vi "monitoring_sys_final.vi"() -> ()   [LabVIEW 2023]
panel:
  in  "?":T1(tab)
  in  "?":bool
  out "Humidity [%]":dbl
  out "Temperture [C] 2":dbl
  out "Oxygen Level [%]":dbl
  out "?":bool
  out "Door's status 2":bool
  out "?":string
  out "string array 2":string[](array[string]) caption="Entry and Exit Data"
  out "Waiting for Message 2":bool
  in  "?":T2(tab)
  out "Pressure Gauge 130B":picture
  out "Glove Box Panel_001 130B":picture
  out "Glove Box Panel_011 130B":picture
  out "Glove Box Panel_002 130B":picture
  out "Glove Box Panel_022 130B":picture
  out "?":bool
  out "Door's status":bool
  out "Oxygen Level [%]":dbl
  out "Temperture [C]":dbl
  out "Humidity [%]":dbl
  out "Waiting for Message":bool
  out "?":string
  in  "?":bool
  out "string array":string[](array[string]) caption="Entry and Exit Data"
  in  "?":bool
  out "Humidity [%]  2":dbl
  out "Temperture [C] 3":dbl
  out "Oxygen Level [%]  2":dbl
  out "?":bool
  out "Waiting for Message 3":bool
  out "Message from Server":string
  out "Error Out":errorcluster caption="Error"
  out "Data from ESP32":dbl[](array[numeric])
  out "Error Out 2":errorcluster caption="Error 2"
  out "Error Out 3":errorcluster caption="Error"
  out "Data from ESP32 2":dbl[](array[numeric])
  out "Data from ESP32 3":dbl[](array[numeric])
  out "Message from Server 2":string
  out "Message from Server 3":string
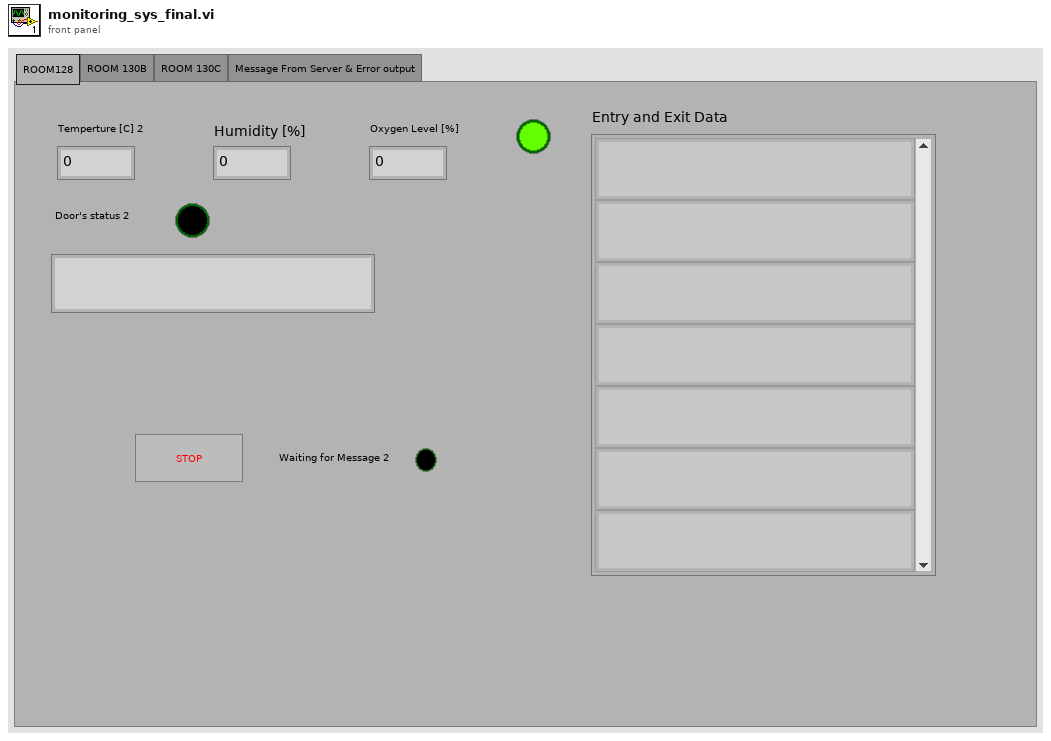
[diagram p1: front panel]
types:
  T1 = enum32{"ROOM128", "ROOM 130B", "ROOM 130C", "Message From Server & Error output"}
  T2 = enum32{"Liquid Nitrogen Tank gauge", "Glove Box 01 Control Panel", "Glove Box 01 Matchine Oil Level", "Glove Box 02 Control Panel", "Glove Box 02 Matchine Oil Level"}
  T3 = enum16{"Standard", "Buffered", "CRLF", "Immediate"}
  T4 = typedef "imagedata.ctl" = cluster{"image type":i32, "image depth":i32, "image":u8[], "mask":u8[], "colors":u32[], "Rectangle":cluster{"left":i16, "top":i16, "right":i16, "bottom":i16}}
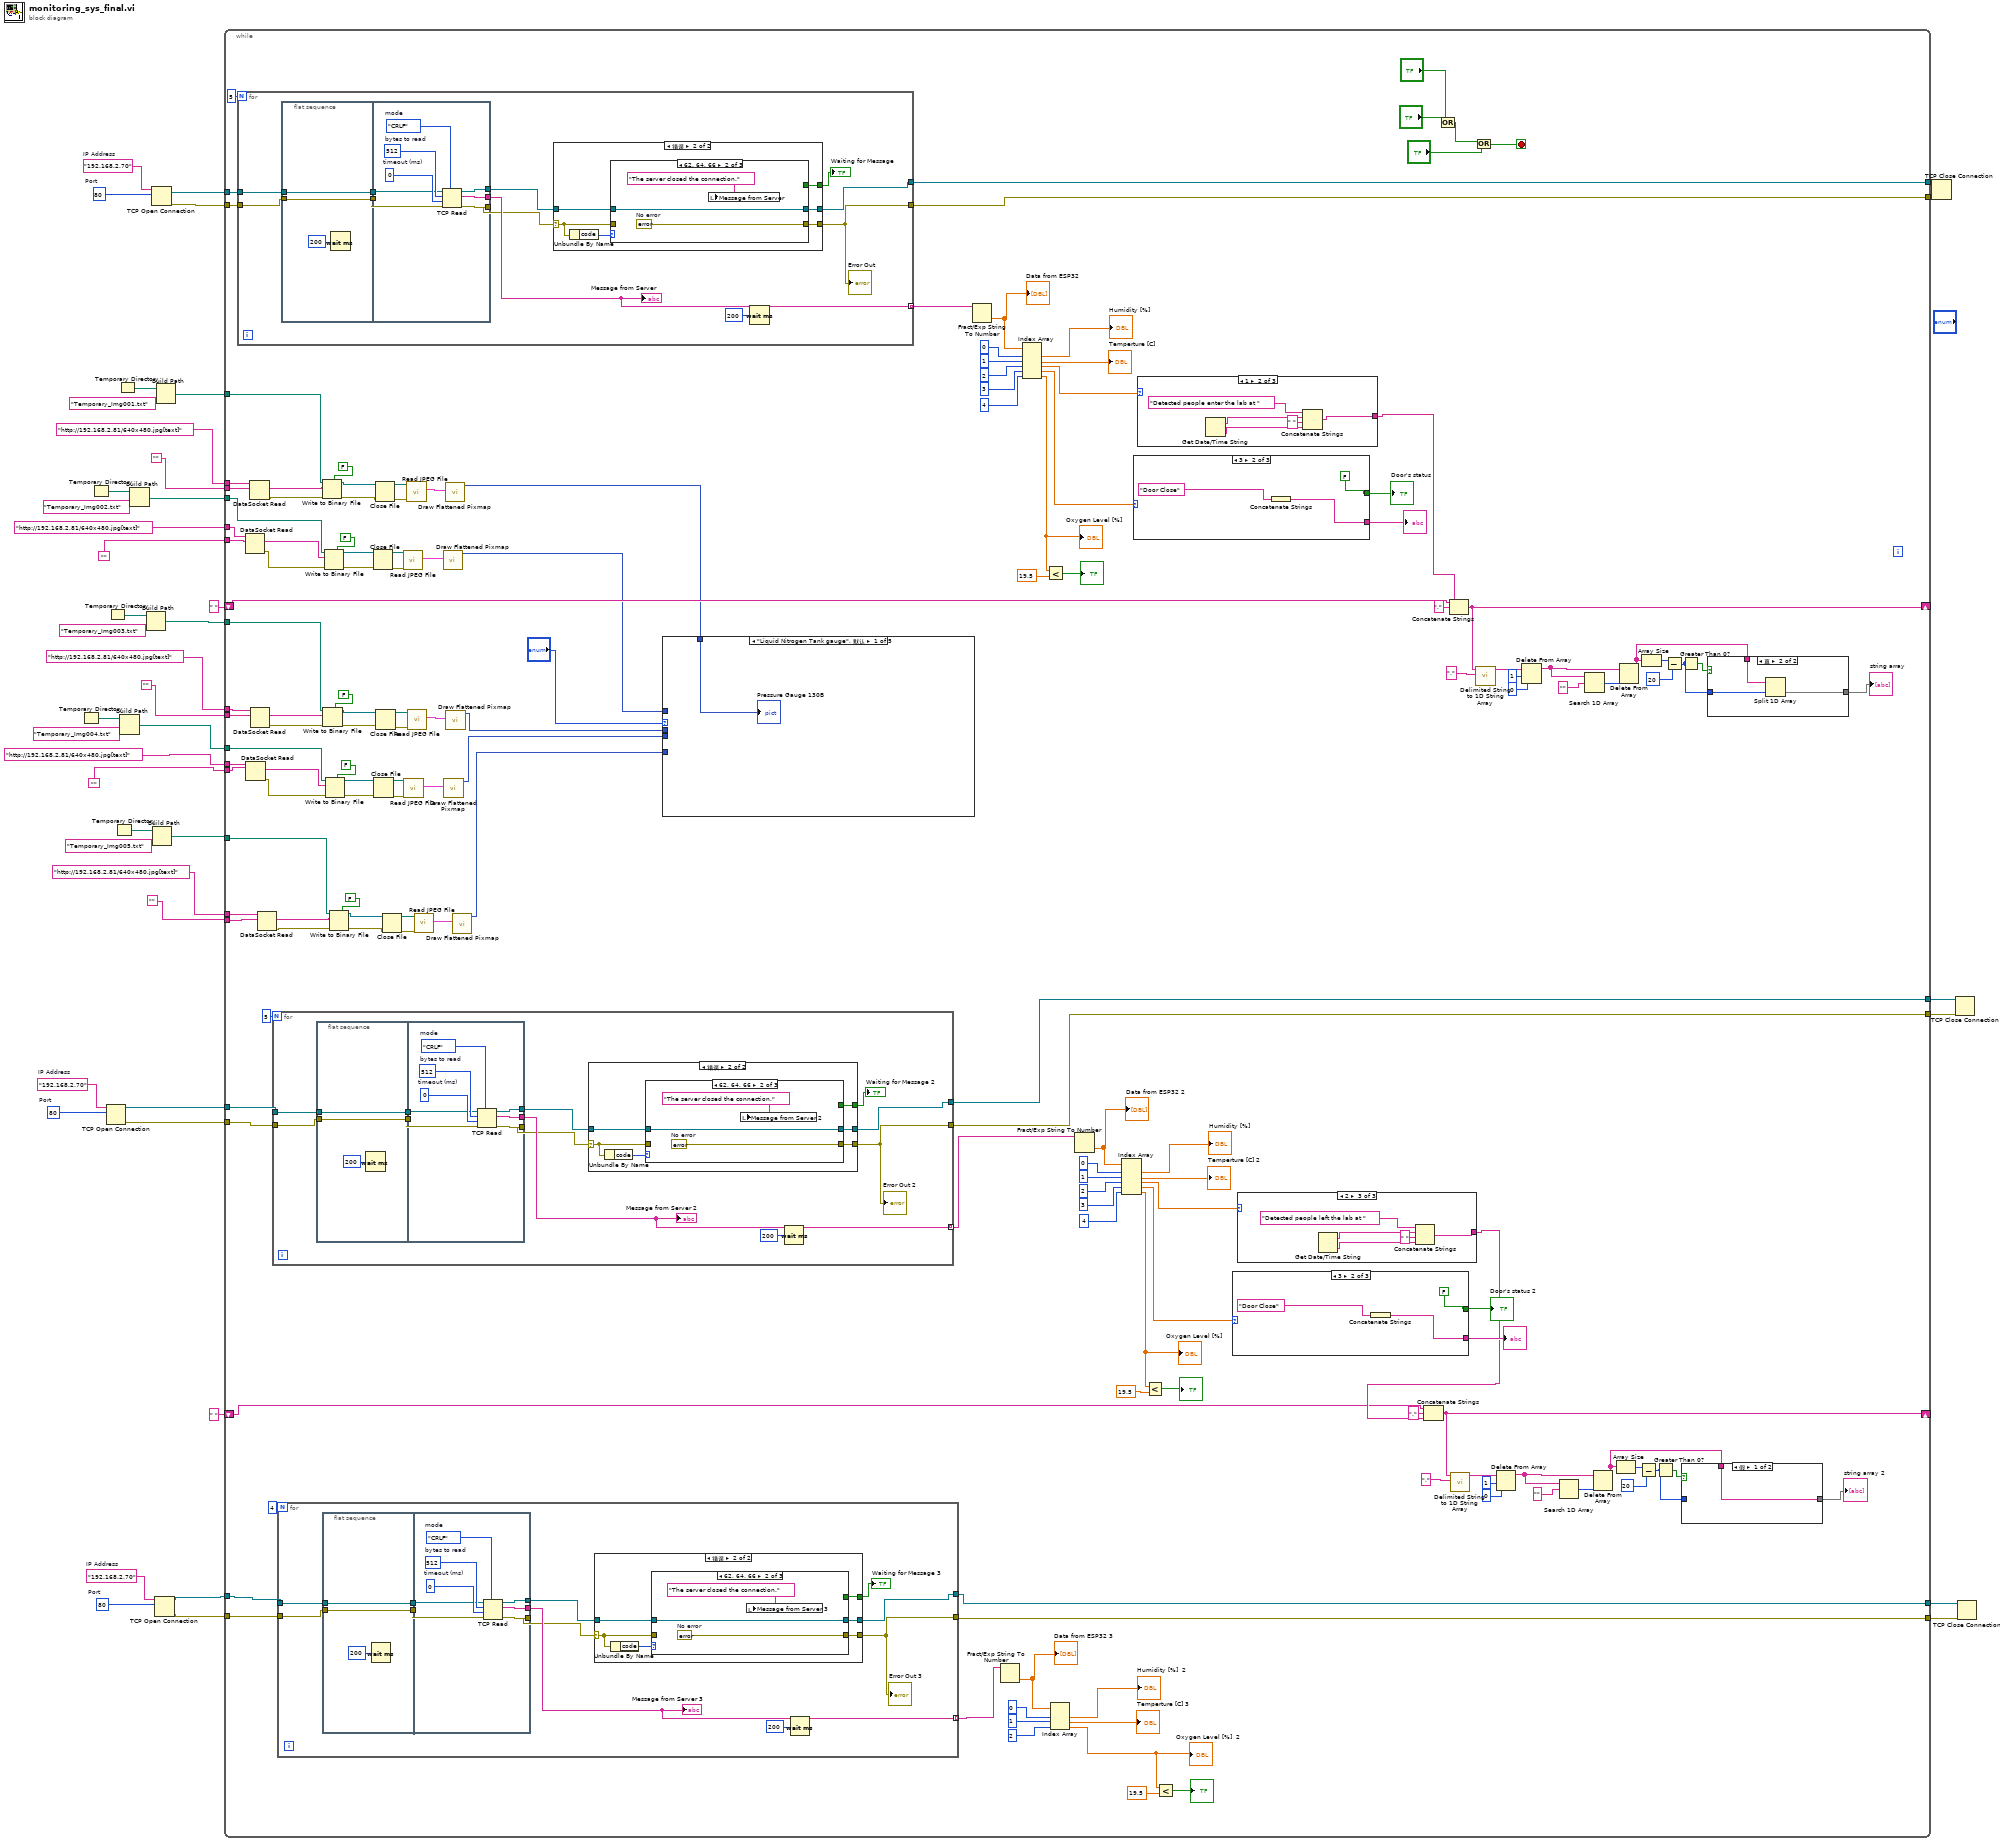
[diagram p0: block diagram]
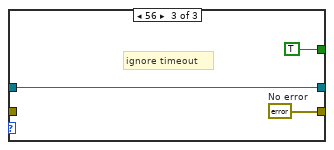
[diagram p4: hidden frame]
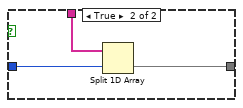
[diagram p5: hidden frame]
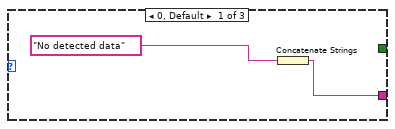
[diagram p6: hidden frame]
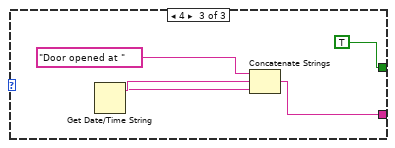
[diagram p7: hidden frame]
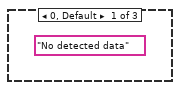
[diagram p8: hidden frame]
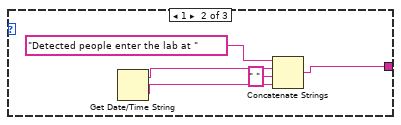
[diagram p9: hidden frame]
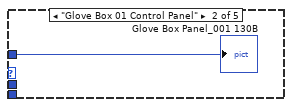
[diagram p10: hidden frame]
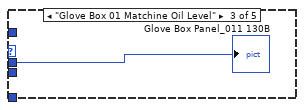
[diagram p11: hidden frame]
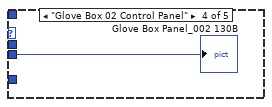
[diagram p12: hidden frame]
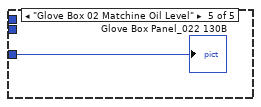
[diagram p13: hidden frame]
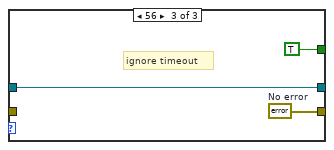
[diagram p16: hidden frame]
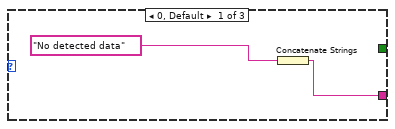
[diagram p18: hidden frame]
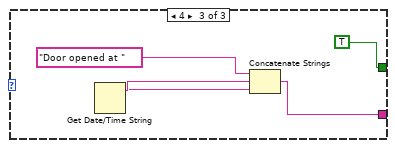
[diagram p19: hidden frame]
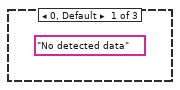
[diagram p20: hidden frame]
diagram:
  w7 = u16 80  # Port
  w8 = "192.168.2.70"  # IP Address
  w28 = u16 80  # Port
  w29 = "192.168.2.70"  # IP Address
  w44 = u16 80  # Port
  w45 = "192.168.2.70"  # IP Address
  n1 = Temporary Directory() -> (w23:path)
  n2 = Temporary Directory() -> (w32:path)
  n3 = TCP Open Connection(address=w29, remote port or service name=w28) -> (connection ID=w27:refnum<k5>, error out=w26:errorcluster)  [unwired: 3 in]
  n4 = Temporary Directory() -> (w25:path)
  n5 = Temporary Directory() -> (w15:path)
  n6 = Temporary Directory() -> (w35:path)
  n7 = Build Path(base path=w23, name or relative path="Temporary_Img004.txt") -> (appended path=w18:path)
  n8 = Build Path(base path=w32, name or relative path="Temporary_Img002.txt") -> (appended path=w30:path)
  n9 = Build Path(base path=w25, name or relative path="Temporary_Img003.txt") -> (appended path=w21:path)
  n10 = TCP Open Connection(address=w45, remote port or service name=w44) -> (connection ID=w43:refnum<k5>, error out=w42:errorcluster)  [unwired: 3 in]
  n11 = Build Path(base path=w15, name or relative path="Temporary_Img005.txt") -> (appended path=w13:path)
  n12 = TCP Open Connection(address=w8, remote port or service name=w7) -> (connection ID=w6:refnum<k5>, error out=w5:errorcluster)  [unwired: 3 in]
  n13 = Build Path(base path=w35, name or relative path="Temporary_Img001.txt") -> (appended path=w33:path)
  n14 = while {
    tunnel: w43 -> [w201]
    tunnel: w42 -> [w200]
    tunnel: [w199] -> w41
    tunnel: [w198] -> w40
    tunnel: "http://192.168.2.81/640x480.jpg[text]" ("URL to JPG Image") -> [w167]
    tunnel: "" -> [w166]
    tunnel: "http://192.168.2.81/640x480.jpg[text]" ("URL to JPG Image") -> [w165]
    tunnel: "" -> [w164]
    shift-right: [w157] -> _
    shift-left: " " -> [w159]
    tunnel: w33 -> [w161]
    tunnel: w30 -> [w160]
    tunnel: w27 -> [w136]
    tunnel: w26 -> [w135]
    tunnel: w21 -> [w118]
    tunnel: "http://192.168.2.81/640x480.jpg[text]" ("URL to JPG Image") -> [w117]
    tunnel: "" -> [w116]
    tunnel: w18 -> [w115]
    tunnel: "http://192.168.2.81/640x480.jpg[text]" ("URL to JPG Image") -> [w114]
    tunnel: "" -> [w113]
    tunnel: w13 -> [w104]
    tunnel: "http://192.168.2.81/640x480.jpg[text]" ("URL to JPG Image") -> [w103]
    tunnel: "" -> [w102]
    shift-right: [w64] -> _
    shift-left: " " -> [w63]
    tunnel: w6 -> [w61]
    tunnel: w5 -> [w60]
    tunnel: [w49] -> w4
    tunnel: [w48] -> w3
    tunnel: [w47] -> w2
    tunnel: [w46] -> w1
    stop <- w177 stop-if-true
    n15 = for {
      N: 5 -> [_]
      tunnel: w201 -> [w340]
      tunnel: w200 -> [w339]
      tunnel: [w333] -> w199
      tunnel: [w332] -> w198
      tunnel: [w337] -> w197 mode=indexing
      n16 = flat-sequence {
        tunnel: w340 -> [w361]
        tunnel: [w361] -> w342
        tunnel: [w360] -> w341
        tunnel: w339 -> [w360]
        tunnel: [w366] -> w336
        tunnel: [w365] -> w337
        tunnel: [w364] -> w335
        tunnel: w342 -> [w363]
        tunnel: w341 -> [w362]
        frame #0 {
          n17 = Wait (ms)(milliseconds to wait=u32 200 ("等待时间（毫秒）")) -> ()  [unwired: 1 out]
        }
        frame #1 {
          w368 = 0  # timeout (ms)
          w369 = T3."CRLF"  # mode
          w367 = 512  # bytes to read
          n18 = TCP Read(connection ID=w363, bytes to read=w367, error in (no error)=w362, 7:w369, 9:w368) -> (connection ID out=w364:refnum<k5>, data out=w365:string, error out=w366:errorcluster)
        }
      }
      n19 = case shown="错误" w336 {
        selector: w336 -> [w344 w349]
        tunnel: [w344 w348] -> w332
        tunnel: w335 -> [w343 w347]
        tunnel: [w343 w346] -> w333
        tunnel: [_ w345] -> w334
        frame No Error {
        }
        frame Error {
          n20 = Unbundle By Name(w349) -> ("code"=w350:i32)
          n21 = case shown="62, 64, 66" w350 {
            tunnel: w349 -> [w352 _ _]
            tunnel: [w352 w355 w358] -> w348
            tunnel: [w351 w354 w357] -> w346
            tunnel: w347 -> [w351 w354 w357]
            tunnel: [_ _ TRUE] -> w345
            frame Default {
            }
            frame 62, 64, 66 {
              w355 = errorcluster {"status"=FALSE, "code"=0, "source"=""}  # No error
              n22 = local write "Message from Server"("The server closed the connection." ("Server Closed")) -> ()
            }
            frame 56 {
              w358 = errorcluster {"status"=FALSE, "code"=0, "source"=""}  # No error
              # "ignore timeout"
            }
          }
        }
      }
      "Waiting for Message" <- w334
      "Error Out" <- w332
      n23 = Wait (ms)(milliseconds to wait=u32 200) -> ()  [unwired: 1 out]
      "Message from Server" <- w337
    }
    n24 = DataSocket Read(10:w166, 11:w167) -> (0:w168:errorcluster, 2:w169:string)  [unwired: 1 in, 7 out]
    n25 = DataSocket Read(10:w113, 11:w114) -> (0:w121:errorcluster, 2:w122:string)  [unwired: 1 in, 7 out]
    n26 = DataSocket Read(10:w164, 11:w165) -> (0:w162:errorcluster, 2:w163:string)  [unwired: 1 in, 7 out]
    n27 = DataSocket Read(10:w116, 11:w117) -> (0:w119:errorcluster, 2:w120:string)  [unwired: 1 in, 7 out]
    n28 = DataSocket Read(10:w102, 11:w103) -> (0:w105:errorcluster, 2:w106:string)  [unwired: 1 in, 7 out]
    n29 = for {
      N: 5 -> [_]
      tunnel: w136 -> [w278]
      tunnel: w135 -> [w277]
      tunnel: [w271] -> w49
      tunnel: [w270] -> w48
      tunnel: [w275] -> w80 mode=indexing
      n30 = flat-sequence {
        tunnel: w278 -> [w299]
        tunnel: [w299] -> w280
        tunnel: [w298] -> w279
        tunnel: w277 -> [w298]
        tunnel: [w304] -> w274
        tunnel: [w303] -> w275
        tunnel: [w302] -> w273
        tunnel: w280 -> [w301]
        tunnel: w279 -> [w300]
        frame #0 {
          n31 = Wait (ms)(milliseconds to wait=u32 200 ("等待时间（毫秒）")) -> ()  [unwired: 1 out]
        }
        frame #1 {
          w306 = 0  # timeout (ms)
          w307 = T3."CRLF"  # mode
          w305 = 512  # bytes to read
          n32 = TCP Read(connection ID=w301, bytes to read=w305, error in (no error)=w300, 7:w307, 9:w306) -> (connection ID out=w302:refnum<k5>, data out=w303:string, error out=w304:errorcluster)
        }
      }
      n33 = case shown="错误" w274 {
        selector: w274 -> [w282 w287]
        tunnel: [w282 w286] -> w270
        tunnel: w273 -> [w281 w285]
        tunnel: [w281 w284] -> w271
        tunnel: [_ w283] -> w272
        frame No Error {
        }
        frame Error {
          n34 = Unbundle By Name(w287) -> ("code"=w288:i32)
          n35 = case shown="62, 64, 66" w288 {
            tunnel: w287 -> [w290 _ _]
            tunnel: [w290 w293 w296] -> w286
            tunnel: [w289 w292 w295] -> w284
            tunnel: w285 -> [w289 w292 w295]
            tunnel: [_ _ TRUE] -> w283
            frame Default {
            }
            frame 62, 64, 66 {
              w293 = errorcluster {"status"=FALSE, "code"=0, "source"=""}  # No error
              n36 = local write "Message from Server 2"("The server closed the connection." ("Server Closed")) -> ()
            }
            frame 56 {
              w296 = errorcluster {"status"=FALSE, "code"=0, "source"=""}  # No error
              # "ignore timeout"
            }
          }
        }
      }
      "Waiting for Message 2" <- w272
      "Error Out 2" <- w270
      n37 = Wait (ms)(milliseconds to wait=u32 200) -> ()  [unwired: 1 out]
      "Message from Server 2" <- w275
    }
    n38 = for {
      N: 4 -> [_]
      tunnel: w61 -> [w211]
      tunnel: w60 -> [w210]
      tunnel: [w204] -> w47
      tunnel: [w203] -> w46
      tunnel: [w208] -> w50 mode=indexing
      n39 = flat-sequence {
        tunnel: w211 -> [w232]
        tunnel: [w232] -> w213
        tunnel: [w231] -> w212
        tunnel: w210 -> [w231]
        tunnel: [w237] -> w207
        tunnel: [w236] -> w208
        tunnel: [w235] -> w206
        tunnel: w213 -> [w234]
        tunnel: w212 -> [w233]
        frame #0 {
          n40 = Wait (ms)(milliseconds to wait=u32 200 ("等待时间（毫秒）")) -> ()  [unwired: 1 out]
        }
        frame #1 {
          w239 = 0  # timeout (ms)
          w240 = T3."CRLF"  # mode
          w238 = 512  # bytes to read
          n41 = TCP Read(connection ID=w234, bytes to read=w238, error in (no error)=w233, 7:w240, 9:w239) -> (connection ID out=w235:refnum<k5>, data out=w236:string, error out=w237:errorcluster)
        }
      }
      n42 = case shown="错误" w207 {
        selector: w207 -> [w215 w220]
        tunnel: [w215 w219] -> w203
        tunnel: w206 -> [w214 w218]
        tunnel: [w214 w217] -> w204
        tunnel: [_ w216] -> w205
        frame No Error {
        }
        frame Error {
          n43 = Unbundle By Name(w220) -> ("code"=w221:i32)
          n44 = case shown="62, 64, 66" w221 {
            tunnel: w220 -> [w223 _ _]
            tunnel: [w223 w226 w229] -> w219
            tunnel: [w222 w225 w228] -> w217
            tunnel: w218 -> [w222 w225 w228]
            tunnel: [_ _ TRUE] -> w216
            frame Default {
            }
            frame 62, 64, 66 {
              w226 = errorcluster {"status"=FALSE, "code"=0, "source"=""}  # No error
              n45 = local write "Message from Server 3"("The server closed the connection." ("Server Closed")) -> ()
            }
            frame 56 {
              w229 = errorcluster {"status"=FALSE, "code"=0, "source"=""}  # No error
              # "ignore timeout"
            }
          }
        }
      }
      "Waiting for Message 3" <- w205
      "Error Out 3" <- w203
      n46 = Wait (ms)(milliseconds to wait=u32 200) -> ()  [unwired: 1 out]
      "Message from Server 3" <- w208
    }
    n47 = Write to Binary File(file (use dialog)=w161, data=w163, error in=w162, 5:FALSE ("prepend array or string size? (T)")) -> (refnum out=w173:refnum<file>, error out=w172:errorcluster)  [unwired: 3 out]
    n48 = Write to Binary File(file (use dialog)=w118, data=w120, error in=w119, 5:FALSE ("prepend array or string size? (T)")) -> (refnum out=w126:refnum<file>, error out=w125:errorcluster)  [unwired: 3 out]
    n49 = Write to Binary File(file (use dialog)=w160, data=w169, error in=w168, 5:FALSE ("prepend array or string size? (T)")) -> (refnum out=w171:refnum<file>, error out=w170:errorcluster)  [unwired: 3 out]
    n50 = Write to Binary File(file (use dialog)=w115, data=w122, error in=w121, 5:FALSE ("prepend array or string size? (T)")) -> (refnum out=w124:refnum<file>, error out=w123:errorcluster)  [unwired: 3 out]
    n51 = Write to Binary File(file (use dialog)=w104, data=w106, error in=w105, 5:FALSE ("prepend array or string size? (T)")) -> (refnum out=w108:refnum<file>, error out=w107:errorcluster)  [unwired: 3 out]
    n52 = Close File(refnum=w171, error in=w170) -> (path=w182:path, error out=w184:errorcluster)
    n53 = Close File(refnum=w124, error in=w123) -> (path=w130:path, error out=w132:errorcluster)
    n54 = Close File(refnum=w173, error in=w172) -> (path=w185:path, error out=w186:errorcluster)
    n55 = Close File(refnum=w126, error in=w125) -> (path=w133:path, error out=w134:errorcluster)
    n56 = Close File(refnum=w108, error in=w107) -> (path=w111:path, error out=w112:errorcluster)
    n57 = call <vilib>:"Read JPEG File.vi"("error in (no error)"=w184, "path to JPEG file"=w182) -> ("image data"=w183:T4)  [unwired: 7 in, 2 out]
    n58 = call <vilib>:"Read JPEG File.vi"("error in (no error)"=w132, "path to JPEG file"=w130) -> ("image data"=w131:T4)  [unwired: 7 in, 2 out]
    n59 = call <vilib>:"Read JPEG File.vi"("error in (no error)"=w186, "path to JPEG file"=w185) -> ("image data"=w176:T4)  [unwired: 9 out]
    n60 = call <vilib>:"Read JPEG File.vi"("error in (no error)"=w134, "path to JPEG file"=w133) -> ("image data"=w129:T4)  [unwired: 9 out]
    n61 = call <vilib>:"Read JPEG File.vi"("error in (no error)"=w112, "path to JPEG file"=w111) -> ("image data"=w110:T4)  [unwired: 9 out]
    n62 = call <vilib>:"Draw Flattened Pixmap.vi"("image data"=w183) -> ("new picture"=w99:picture)  [unwired: 1 in, 7 out]
    n63 = call <vilib>:"Draw Flattened Pixmap.vi"("image data"=w131) -> ("new picture"=w97:picture)  [unwired: 1 in, 7 out]
    n64 = call <vilib>:"Draw Flattened Pixmap.vi"("image data"=w176) -> ("new picture"=w100:picture)  [unwired: 1 in, 7 out]
    n65 = call <vilib>:"Draw Flattened Pixmap.vi"("image data"=w129) -> ("new picture"=w98:picture)  [unwired: 1 in, 7 out]
    n66 = call <vilib>:"Draw Flattened Pixmap.vi"("image data"=w110) -> ("new picture"=w96:picture)  [unwired: 1 in, 7 out]
    n67 = case shown="\"Liquid Nitrogen Tank gauge\", 默认" "?" {
      tunnel: w100 -> [w265 _ _ _ _]
      tunnel: w99 -> [_ w266 _ _ _]
      tunnel: w98 -> [_ _ w267 _ _]
      tunnel: w97 -> [_ _ _ w268 _]
      tunnel: w96 -> [_ _ _ _ w269]
      frame "Liquid Nitrogen Tank gauge", Default {
        "Pressure Gauge 130B" <- w265
      }
      frame "Glove Box 01 Control Panel" {
        "Glove Box Panel_001 130B" <- w266
      }
      frame "Glove Box 01 Matchine Oil Level" {
        "Glove Box Panel_011 130B" <- w267
      }
      frame "Glove Box 02 Control Panel" {
        "Glove Box Panel_002 130B" <- w268
      }
      frame "Glove Box 02 Matchine Oil Level" {
        "Glove Box Panel_022 130B" <- w269
      }
    }
    n68 = Fract/Exp String To Number(string=w197) -> (number=w194:dbl[])  [unwired: 3 in, 1 out]
    "Data from ESP32" <- w194
    n69 = Fract/Exp String To Number(string=w50) -> (number=w57:dbl[])  [unwired: 3 in, 1 out]
    "Data from ESP32 3" <- w57
    n70 = Index Array(array=w194, index #1=0 ("索引"), index #2=1 ("索引"), index #3=2 ("索引"), index #4=3 ("索引"), index #5=4 ("索引")) -> (element #1=→"Humidity [%]":dbl, element #2=→"Temperture [C]":dbl, element #3=w189:dbl, element #4=w188:dbl, element #5=w138:dbl)
    "Oxygen Level [%]" <- w138
    n71 = Less?(x=w138, y=19.5) -> (x < y?=→"?":bool)
    n72 = Index Array(array=w57, index #1=0 ("索引"), index #2=1 ("索引"), index #3=2 ("索引")) -> (element #1=→"Humidity [%]  2":dbl, element #2=→"Temperture [C] 3":dbl, element #3=w51:dbl)
    "Oxygen Level [%]  2" <- w51
    n73 = Fract/Exp String To Number(string=w80) -> (number=w93:dbl[])  [unwired: 3 in, 1 out]
    "Data from ESP32 2" <- w93
    n74 = Index Array(array=w93, index #1=0 ("索引"), index #2=1 ("索引"), index #3=2 ("索引"), index #4=3 ("索引"), index #5=4 ("索引")) -> (element #1=→"Humidity [%]":dbl, element #2=→"Temperture [C] 2":dbl, element #3=w88:dbl, element #4=w87:dbl, element #5=w81:dbl)
    "Oxygen Level [%]" <- w81
    n75 = case shown="3" w188 {
      tunnel: [_ FALSE TRUE] -> w187
      tunnel: [w312 w314 w317] -> w158
      frame 0, Default {
        n76 = Concatenate Strings("No detected data") -> (w312:string)
      }
      frame 3 {
        n77 = Concatenate Strings("Door Close") -> (w314:string)
      }
      frame 4 {
        n78 = Get Date/Time String() -> (date string=w321:string, time string=w320:string)  [unwired: 3 in]
        n79 = Concatenate Strings("Door opened at ", w321, w320) -> (w317:string)
      }
    }
    "Door's status" <- w187
    "?" <- w158
    n80 = case shown="1" w189 {
      tunnel: [_ w324 w329] -> w155
      frame 0, Default {
        (unwired) "No detected data"
      }
      frame 1 {
        n81 = Get Date/Time String() -> (date string=w325:string, time string=w323:string)  [unwired: 3 in]
        n82 = Concatenate Strings("Detected people enter the lab at ", w325, " " ("字符串"), w323) -> (w324:string)
      }
      frame 2 {
        n83 = Get Date/Time String() -> (date string=w331:string, time string=w328:string)  [unwired: 3 in]
        n84 = Concatenate Strings("Detected people left the lab at ", w331, " " ("字符串"), w328) -> (w329:string)
      }
    }
    n85 = Less?(x=w81, y=19.5) -> (x < y?=→"?":bool)
    n86 = Less?(x=w51, y=19.5) -> (x < y?=→"?":bool)
    n87 = case shown="3" w87 {
      tunnel: [_ FALSE TRUE] -> w86
      tunnel: [w245 w247 w250] -> w85
      frame 0, Default {
        n88 = Concatenate Strings("No detected data") -> (w245:string)
      }
      frame 3 {
        n89 = Concatenate Strings("Door Close") -> (w247:string)
      }
      frame 4 {
        n90 = Get Date/Time String() -> (date string=w254:string, time string=w253:string)  [unwired: 3 in]
        n91 = Concatenate Strings("Door opened at ", w254, w253) -> (w250:string)
      }
    }
    "Door's status 2" <- w86
    "?" <- w85
    n92 = case shown="2" w88 {
      tunnel: [_ w257 w262] -> w65
      frame 0, Default {
        (unwired) "No detected data"
      }
      frame 1 {
        n93 = Get Date/Time String() -> (date string=w258:string, time string=w256:string)  [unwired: 3 in]
        n94 = Concatenate Strings("Detected people enter the lab at ", w258, " " ("字符串"), w256) -> (w257:string)
      }
      frame 2 {
        n95 = Get Date/Time String() -> (date string=w264:string, time string=w261:string)  [unwired: 3 in]
        n96 = Concatenate Strings("Detected people left the lab at ", w264, " " ("字符串"), w261) -> (w262:string)
      }
    }
    n97 = Concatenate Strings(w63, "," ("字符串"), w65) -> (w64:string)
    n98 = Or(x="?", y="?") -> (x .or. y?=w179:bool)
    n99 = Concatenate Strings(w159, "," ("字符串"), w155) -> (w157:string)
    n100 = call <vilib>:"Delimited String to 1D String Array.vi"("delimiter"=",", "delimited string"=w64) -> ("string array"=w77:string[])  [unwired: 9 in]
    n101 = Or(x=w179, y="?") -> (x .or. y?=w177:bool)
    n102 = call <vilib>:"Delimited String to 1D String Array.vi"("delimiter"=",", "delimited string"=w157) -> ("string array"=w153:string[])  [unwired: 9 in]
    n103 = Delete From Array(array=w77, length=1 ("长度"), index=0 ("索引")) -> (array with subset deleted=w73:string[])  [unwired: 1 out]
    n104 = Delete From Array(array=w153, length=1 ("长度"), index=0 ("索引")) -> (array with subset deleted=w149:string[])  [unwired: 1 out]
    n105 = Search 1D Array(1D array=w73, element="" ("元素")) -> (index of element=w72:i32)  [unwired: 1 in]
    n106 = Search 1D Array(1D array=w149, element="" ("元素")) -> (index of element=w148:i32)  [unwired: 1 in]
    n107 = Delete From Array(array=w73, index=w72) -> (array with subset deleted=w68:string[])  [unwired: 1 in, 1 out]
    n108 = Array Size(array=w68) -> (size(s)=w71:i32)
    n109 = Delete From Array(array=w149, index=w148) -> (array with subset deleted=w144:string[])  [unwired: 1 in, 1 out]
    n110 = Subtract(x=w71, y=20) -> (x-y=w67:i32)
    n111 = Array Size(array=w144) -> (size(s)=w147:i32)
    n112 = Greater Than 0?(x=w67) -> (x > 0?=w69:bool)
    n113 = Subtract(x=w147, y=20) -> (x-y=w143:i32)
    n114 = Greater Than 0?(x=w143) -> (x > 0?=w145:bool)
    n115 = case shown="假" w69 {
      tunnel: w68 -> [w241 w244]
      tunnel: w67 -> [_ w243]
      tunnel: [w241 w242] -> w66
      frame False {
      }
      frame True {
        n116 = Split 1D Array(array=w244, index=w243) -> (second subarray=w242:string[])  [unwired: 1 out]
      }
    }
    "string array 2" <- w66
    n117 = case shown="真" w145 {
      tunnel: w144 -> [w308 w311]
      tunnel: w143 -> [_ w310]
      tunnel: [w308 w309] -> w142
      frame False {
      }
      frame True {
        n118 = Split 1D Array(array=w311, index=w310) -> (second subarray=w309:string[])  [unwired: 1 out]
      }
    }
    "string array" <- w142
  }
  n119 = TCP Close Connection(connection ID=w41, error in (no error)=w40) -> ()  [unwired: 3 out]
  n120 = TCP Close Connection(connection ID=w4, error in (no error)=w3) -> ()  [unwired: 3 out]
  n121 = TCP Close Connection(connection ID=w2, error in (no error)=w1) -> ()  [unwired: 3 out]
